vi "xio.copy_lua.vi"(5 "LuaVIEW reference":T1) -> (15 "error out":errorcluster)   [LabVIEW 2012]
doc: "Copies the file or directory specified by the source path to the target path.\nParameters:\nstr:source, path of file or directory to copy\nstr:taget, path to copy to\nErrors:\nFile or directory not found.\nFile in use.\nAccess denied.\nDisk full."
uses:
  typedefs/t_LuaVIEW Reference.ctl
  subvis/private/LuaVIEW Pull (path).vi
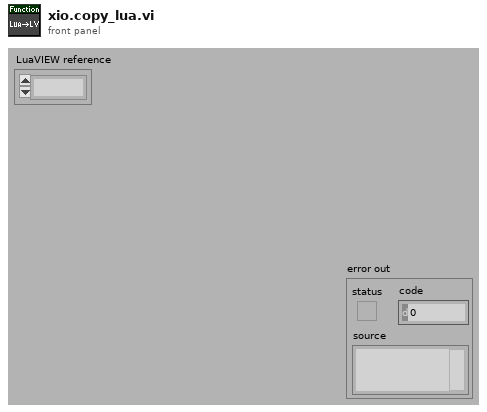
[diagram p1: front panel]
types:
  T1 = typedef "t_LuaVIEW Reference.ctl" = refnum<k1>
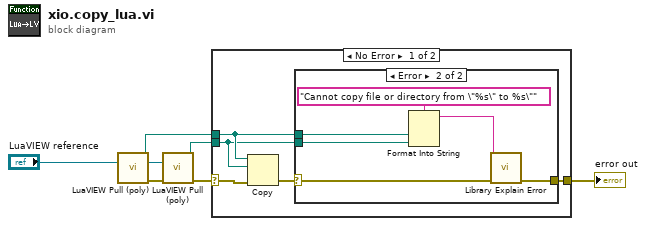
[diagram p0: block diagram]
diagram:
  n1 = call-poly "LuaVIEW Pull (poly).vi"("LuaVIEW reference in"="LuaVIEW reference") -> ("path"=w6:path, "LuaVIEW reference out"=w4:T1, "error out"=w5:errorcluster)  [unwired: 12 in]
  n2 = call-poly "LuaVIEW Pull (poly).vi"("LuaVIEW reference in"=w4, "error in (no error)"=w5) -> ("path"=w3:path, "error out"=w2:errorcluster)  [unwired: 11 in, 1 out]
  n3 = case shown="No Error" w2 {
    selector: w2 -> [w12 w20]
    tunnel: w6 -> [w9 _]
    tunnel: w3 -> [w8 _]
    tunnel: [w10 w20] -> w1
    frame No Error {
      n4 = Copy(8:w12, 10:w8, 11:w9) -> (0:w11:errorcluster)  [unwired: 2 in, 2 out]
      n5 = case shown="Error" w11 {
        selector: w11 -> [w13 w19]
        tunnel: [w13 w18] -> w10
        tunnel: w9 -> [_ w17]
        tunnel: w8 -> [_ w15]
        frame No Error {
        }
        frame Error {
          n6 = Format Into String(format string="Cannot copy file or directory from \"%s\" to %s\"", w17, w15) -> (resulting string=w16:string)  [unwired: 2 in, 1 out]
          n7 = call "Library Explain Error.vi"("explanation prefix (none)"=w16, "error in (no error)"=w19) -> ("explained error"=w18:errorcluster)  [unwired: 13 in]
        }
      }
    }
    frame Error {
    }
  }
  "error out" <- w1
